vi "RFmxSpecAn Get Results Guts(Harms).vi"(0 "Refnum in":T2, 1 "Spectrum in":refnum<vi>, 2 "Marker Freq":refnum<vi>, 3 "Marker Level":refnum<vi>, 5 "Center Freq (Hz)":dbl, 11 "error in (no error)":errorcluster) -> (4 "Refnum out":T2, 6 "Peak Frequency (Hz)":dbl format="%.6p", 8 "Peak Amplitude":dbl format="%.2f", 15 "error out":errorcluster)   [LabVIEW 2018]
uses:
  <vilib>/RFmx/RFInstr/mx/Support/RFmxInstrSupport.llb/niRFmx Instrument Handle.ctl
  <vilib>/RFmx/SpecAn/mx/RFmxSpecAn.llb/RFmxSpecAn Spectrum Fetch Spectrum.vi
  <vilib>/RFmx/SpecAn/mx/RFmxSpecAn.llb/RFmxSpecAn Spectrum Fetch Measurement.vi
  <resource>/objmgr/RFmxSpecAn.rc
  <resource>/objmgr/RFmxInstr.rc
panel:
  out "Status":T1
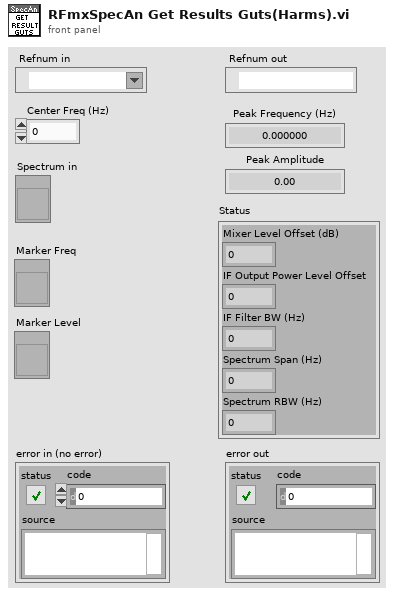
[diagram p1: front panel]
types:
  T1 = cluster{"Mixer Level Offset (dB)":dbl, "IF Output Power Level Offset":dbl, "IF Filter BW (Hz)":dbl, "Spectrum Span (Hz)":dbl, "Spectrum RBW (Hz)":dbl}
  T2 = typedef "niRFmx Instrument Handle.ctl" = refnum<k21>
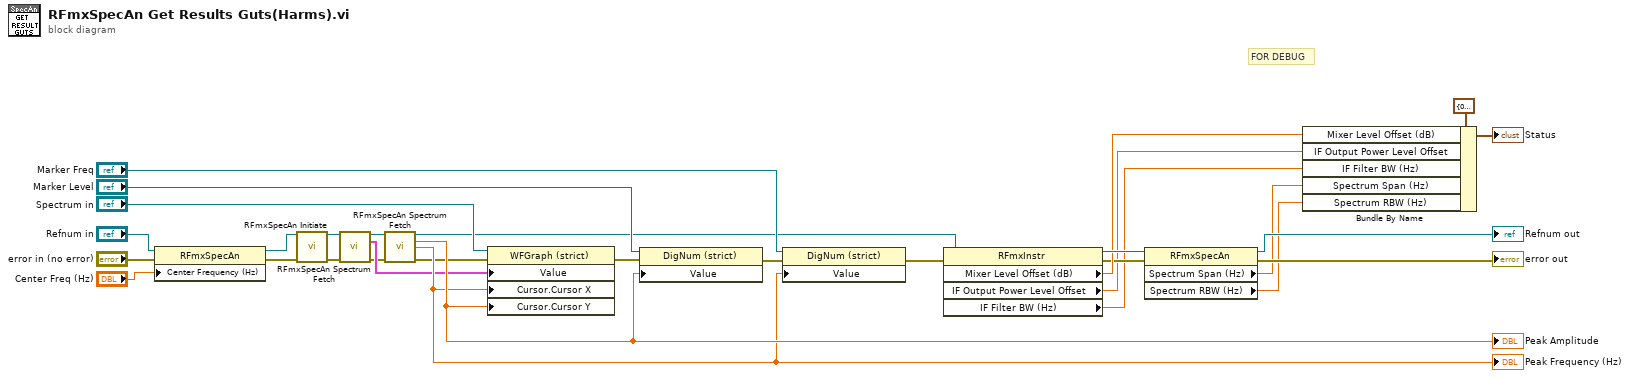
[diagram p0: block diagram]
diagram:
  # "FOR DEBUG"
  n1 = property class="RFmxSpecAn"(reference="Refnum in", error in="error in (no error)", "Center Frequency (Hz)"="Center Freq (Hz)") -> (reference out=w17:T2, error out=w16:errorcluster)
  n2 = call <vilib>:"RFmxSpecAn Initiate.vi"("Instrument Handle In"=w17, "error in (no error)"=w16) -> ("Instrument Handle Out"=w14:refnum<k21>, "error out"=w15:errorcluster)  [unwired: 11 in, 1 out]
  n3 = call-poly <vilib>:"RFmxSpecAn Spectrum Fetch.vi"("Instrument Handle In"=w14, "error in (no error)"=w15) -> ("Instrument Handle Out"=w22:refnum<k21>, "Spectrum"=w25:cluster{"x0":dbl, "dx":dbl, "y":sgl[]}, "error out"=w21:errorcluster)  [unwired: 11 in]
  n4 = call-poly <vilib>:"RFmxSpecAn Spectrum Fetch.vi"("Instrument Handle In"=w22, "error in (no error)"=w21) -> ("Instrument Handle Out"=w12:refnum<k21>, "Peak Amplitude"=w31:dbl, "Peak Frequency (Hz)"=w30:dbl, "error out"=w24:errorcluster)  [unwired: 9 in, 1 out]
  "Peak Frequency (Hz)" <- w30
  "Peak Amplitude" <- w31
  n5 = property class="WFGraph (strict)"(reference="Spectrum in", error in=w24, "Value"=w25, "Cursor.Cursor X"=w30, "Cursor.Cursor Y"=w31) -> (error out=w26:errorcluster)  [unwired: 1 out]
  n6 = property class="DigNum (strict)"(reference="Marker Level", error in=w26, "Value"=w31) -> (error out=w27:errorcluster)  [unwired: 1 out]
  n7 = property class="DigNum (strict)"(reference="Marker Freq", error in=w27, "Value"=w30) -> (error out=w13:errorcluster)  [unwired: 1 out]
  n8 = property class="RFmxInstr"(reference=w12, error in=w13) -> (reference out=w11:refnum<k21>, error out=w5:errorcluster, "Mixer Level Offset (dB)"=w6:dbl, "IF Output Power Level Offset"=w4:dbl, "IF Filter BW (Hz)"=w3:dbl)
  n9 = property class="RFmxSpecAn"(reference=w11, error in=w5) -> (reference out=→"Refnum out":refnum<k21>, error out=→"error out":errorcluster, "Spectrum Span (Hz)"=w2:dbl, "Spectrum RBW (Hz)"=w1:dbl)
  n10 = Bundle By Name(cluster=T1 {"Mixer Level Offset (dB)"=0.0, "IF Output Power Level Offset"=0.0, "IF Filter BW (Hz)"=0.0, "Spectrum Span (Hz)"=0.0, "Spectrum RBW (Hz)"=0.0} ("Status"), "Mixer Level Offset (dB)"=w6, "IF Output Power Level Offset"=w4, "IF Filter BW (Hz)"=w3, "Spectrum Span (Hz)"=w2, "Spectrum RBW (Hz)"=w1) -> (→"Status":T1)
